vi "190624_Simulation_PDFF.vi"() -> ()   [LabVIEW 2019]
uses:
  <vilib>/Utility/Variable/NI_VariableUtilities.lvlib
panel:
  out "all time(s)":dbl
  out "Time slots (sec)":dbl[](array[numeric]) format="%#.10f"
  in  "Sample Rate (Hz)":dbl=1000.0 format="%#_13g"
  in  "STOP":bool
  in  "Load":bool
  in  "CLEAR":bool
  in  "RUN":bool
  out "RMS  X (um)":dbl format="%0.2f"
  out "MAX  X (um)":dbl format="%0.2f"
  out "RMS (one) X (um)":dbl format="%0.2f"
  out "Output X (mm)":dbl[](graph)
  out "CMD X (mm)":dbl[](graph)
  out "Position Error X (um)":dbl[](graph)
  out "Position Command X (mm)":dbl[](graph)
  out "time length":i32=15000
  out "start time":i32=7500
  out "RMS (one) Z (um)":dbl format="%0.2f"
  out "MAX  Z (um)":dbl format="%0.2f"
  out "RMS  Z (um)":dbl format="%0.2f"
  out "Position Error Z (um)":dbl[](graph)
  out "CMD Z (mm)":dbl[](graph)
  out "Output Z (mm)":dbl[](graph)
  out "Position Command Z (mm)":dbl[](graph)
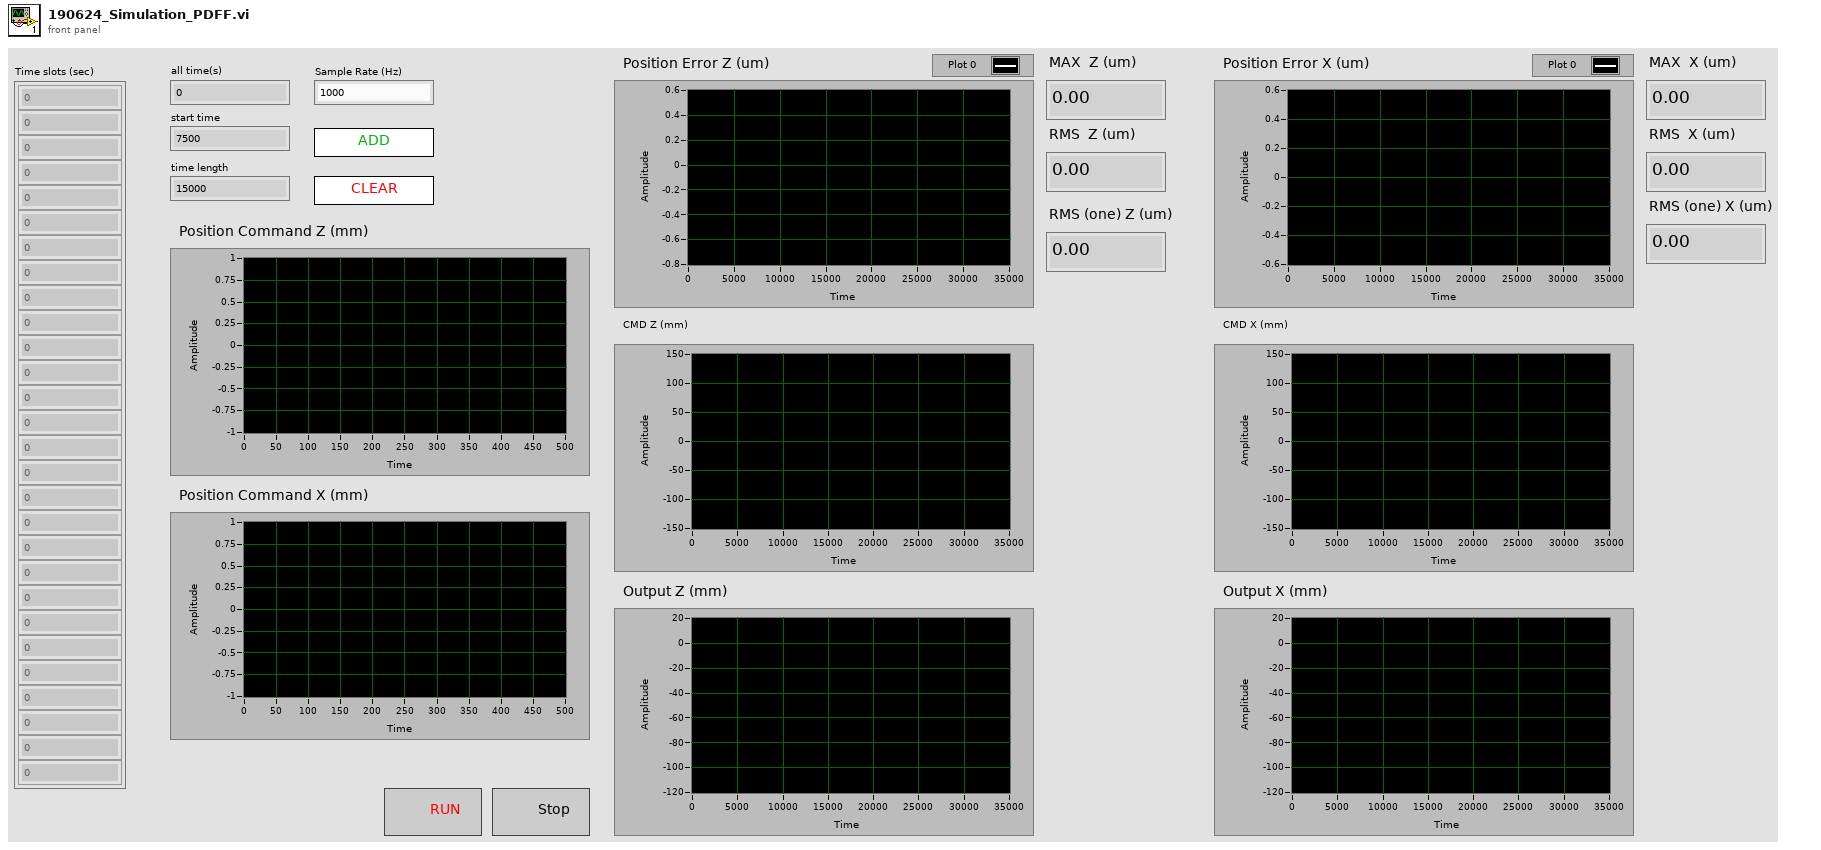
[diagram p1: front panel]
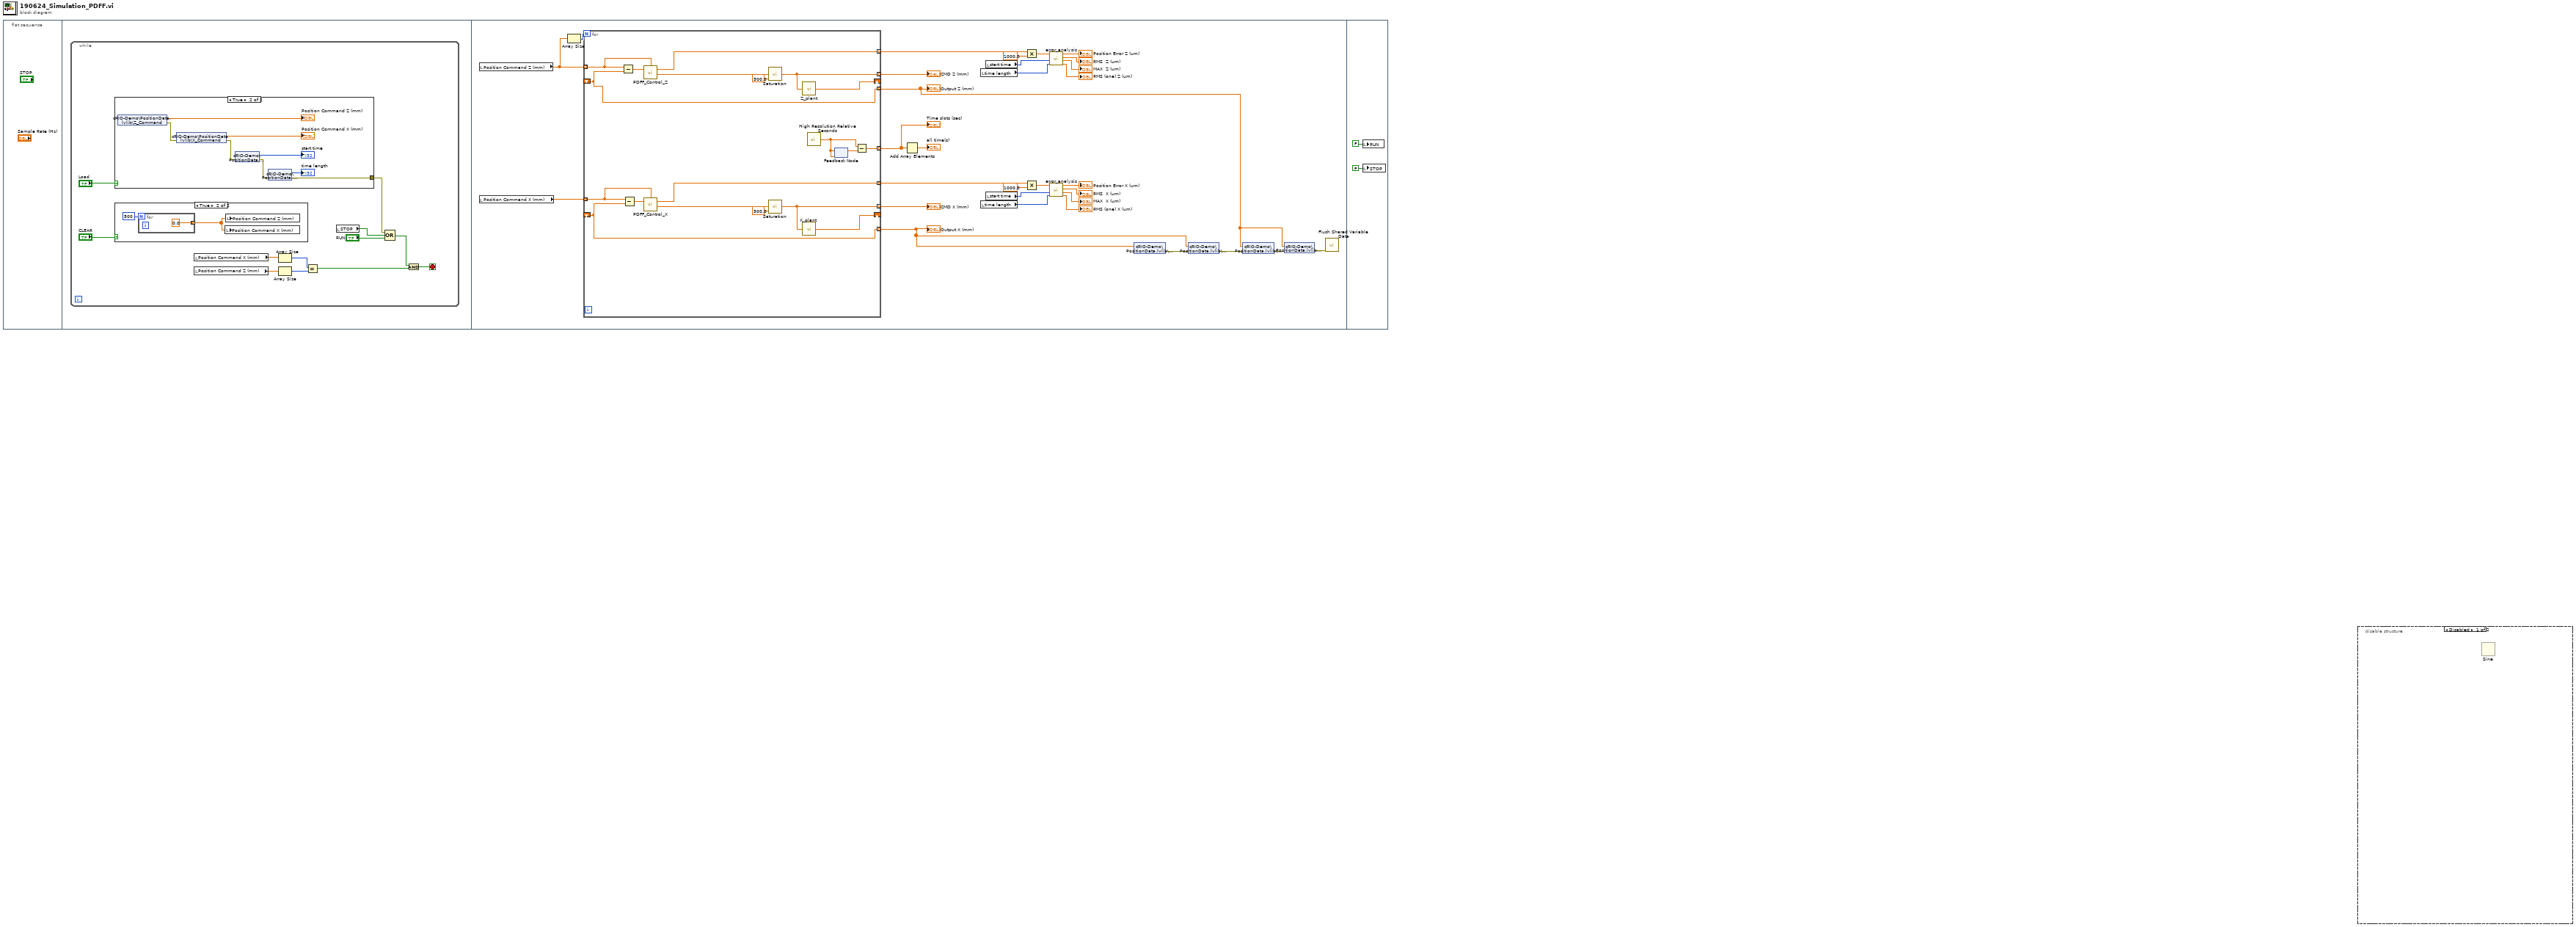
[diagram p0: block diagram]
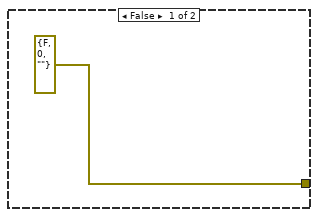
[diagram p3: hidden frame]
diagram:
  n1 = flat-sequence {
    frame #0 {
    }
    frame #1 {
      n2 = while {
        stop <- w9 stop-if-true
        n3 = case shown="True" "Load" {
          tunnel: [errorcluster {"status"=FALSE, "code"=0, "source"=""} ("error IO") w19] -> w1
          frame False {
          }
          frame True {
            n4 = shared-variable "cRIO-Demo\\PositionData.lvlib\\Z_Command"() -> (→"Position Command Z (mm)":dbl[], error out=w22:errorcluster)  [unwired: 1 in]
            n5 = shared-variable "cRIO-Demo\\PositionData.lvlib\\X_Command"(error in=w22) -> (→"Position Command X (mm)":dbl[], error out=w20:errorcluster)
            n6 = shared-variable "cRIO-Demo\\PositionData.lvlib\\t0"(error in=w20) -> (→"start time":i32, error out=w21:errorcluster)
            n7 = shared-variable "cRIO-Demo\\PositionData.lvlib\\tL"(error in=w21) -> (→"time length":i32, error out=w19:errorcluster)
          }
        }
        n8 = case shown="True" "CLEAR" {
          frame False {
          }
          frame True {
            n9 = for {
              N: 500 -> [_]
              tunnel: [0.0 ("element")] -> w14 mode=indexing
            }
            n10 = local write "Position Command X (mm)"(w14) -> ()
            n11 = local write "Position Command Z (mm)"(w14) -> ()
          }
        }
        n12 = local read "Position Command X (mm)"() -> (w10:dbl[])
        n13 = local read "Position Command Z (mm)"() -> (w11:dbl[])
        n14 = Array Size(array=w11) -> (size(s)=w7:i32)
        n15 = Array Size(array=w10) -> (size(s)=w8:i32)
        n16 = Equal?(x=w8, y=w7) -> (x = y?=w6:bool)
        n17 = local read "STOP"() -> (w2:bool)
        n18 = Compound Arithmetic op=OR(w1, w2, "RUN") -> (w4:bool)
        n19 = And(x=w4, y=w6) -> (x .and. y?=w9:bool)
      }
    }
    frame #2 {
      n20 = local read "Position Command Z (mm)"() -> (w54:dbl[])
      n21 = local read "Position Command X (mm)"() -> (w38:dbl[])
      n22 = Array Size(array=w54) -> (size(s)=w53:i32)
      n23 = for {
        N: w53 -> [_]
        shift-right: [w68] -> _
        shift-left: _ -> [w56]
        tunnel: [w56] -> w26 mode=indexing
        tunnel: [w63] -> w34 mode=indexing
        tunnel: [w67] -> w55 mode=indexing
        tunnel: w54 -> [w64] mode=indexing
        tunnel: w38 -> [w61] mode=indexing
        shift-right: [w69] -> _
        shift-left: _ -> [w57]
        tunnel: [w70] -> w37 mode=indexing
        tunnel: [w60] -> w32 mode=indexing
        tunnel: [w57] -> w27 mode=indexing
        tunnel: [w71] -> w36 mode=indexing
        n24 = Subtract(x=w64, y=w56) -> (x-y=w65:dbl)
        n25 = Subtract(x=w61, y=w57) -> (x-y=w58:dbl)
        n26 = call "PDFF_Control_Z.vi"("e(k)"=w65, "r(k)"=w64) -> ("u(k)"=w62:dbl, "e(k)"=w63:dbl)  [unwired: 4 in]
        n27 = call "PDFF_Control_X.vi"("e(k)"=w58, "r(k)"=w61) -> ("u(k)"=w59:dbl, "e(k)"=w60:dbl)  [unwired: 4 in]
        n28 = call "Saturation.vi"("Vmax"=300.0, "uk"=w62) -> ("real uk"=w67:dbl)  [unwired: 3 in]
        n29 = call "Saturation.vi"("Vmax"=300.0, "uk"=w59) -> ("real uk"=w70:dbl)  [unwired: 3 in]
        n30 = call "Z_plant.vi"("u"=w67) -> ("y"=w68:dbl)  [unwired: 4 in]
        n31 = call "X_plant.vi"("u"=w70) -> ("y"=w69:dbl)  [unwired: 4 in]
        n32 = call <vilib>:"High Resolution Relative Seconds.vi"() -> ("relative seconds"=w66:dbl)
        n33 = feedback #1(w66) -> (w72:dbl)
        n34 = feedback-in #1(w66) -> ()
        n35 = Subtract(x=w66, y=w72) -> (x-y=w71:dbl)
      }
      "Output Z (mm)" <- w26
      "CMD Z (mm)" <- w55
      "Output X (mm)" <- w27
      "CMD X (mm)" <- w37
      "Time slots (sec)" <- w36
      n36 = Add Array Elements(numeric array=w36) -> (sum=→"all time(s)":dbl)
      n37 = local read "time length"() -> (w48:i32)
      n38 = local read "time length"() -> (w42:i32)
      n39 = local read "start time"() -> (w47:i32)
      n40 = local read "start time"() -> (w41:i32)
      n41 = Multiply(x=w34, y=1000.0) -> (x*y=w46:dbl[])
      n42 = Multiply(x=w32, y=1000.0) -> (x*y=w39:dbl[])
      n43 = call "error_analysis.vi"("tLength"=w48, "t0"=w47, "data in (um)"=w46) -> ("rms (one) (um)"=→"RMS (one) Z (um)":dbl, "max err (um)"=→"MAX  Z (um)":dbl, "rms (all) (um)"=→"RMS  Z (um)":dbl, "data out (um)"=→"Position Error Z (um)":dbl[])  [unwired: 5 in]
      n44 = call "error_analysis.vi"("tLength"=w42, "t0"=w41, "data in (um)"=w39) -> ("rms (one) (um)"=→"RMS (one) X (um)":dbl, "max err (um)"=→"MAX  X (um)":dbl, "rms (all) (um)"=→"RMS  X (um)":dbl, "data out (um)"=→"Position Error X (um)":dbl[])  [unwired: 5 in]
      n45 = shared-variable "cRIO-Demo\\PositionData.lvlib\\X_EN"(w27) -> (error out=w29:errorcluster)  [unwired: 1 in]
      n46 = shared-variable "cRIO-Demo\\PositionData.lvlib\\X_LS"(w27, error in=w29) -> (error out=w28:errorcluster)
      n47 = shared-variable "cRIO-Demo\\PositionData.lvlib\\Z_EN"(w26, error in=w28) -> (error out=w30:errorcluster)
      n48 = shared-variable "cRIO-Demo\\PositionData.lvlib\\Z_LS"(w26, error in=w30) -> (error out=w25:errorcluster)
      n49 = call <vilib>:"Flush Shared Variable Data.vi"("error in (no error)"=w25) -> ()  [unwired: 10 in, 1 out]
    }
    frame #3 {
      n50 = local write "RUN"(FALSE ("RUN")) -> ()
      n51 = local write "STOP"(FALSE ("STOP")) -> ()
    }
  }
  n52 = disable-structure shown="Disabled" {
    frame Disabled {
      n53 = Sine() -> ()  [unwired: 1 in, 1 out]
    }
    frame Enabled {
    }
  }
